vi "FFT-Rotate.vi"() -> ()   [LabVIEW 2014]
doc: "Use this template to build a VI to use as a subVI."
uses:
  <vilib>/vision/NI_Vision_Development_Module.lvlib
panel:
  out "IF(u,v)I 3":T1(plugin-control)
  out "IF(u,v)I 2":T1(plugin-control)
  out "Rotated":T1(plugin-control)
  out "IF(u,v)I":T1(plugin-control)
  out "Src":T1(plugin-control)
  # ":: MVi Framework V1.0 ::\nAuthor:Gaoke Yang\nEmail: gaoke.yang@yahoo.com\nWeb: www.mvicontrol.com\nCopyright (C) 2015, MVI Technologies All Rights Reserved"
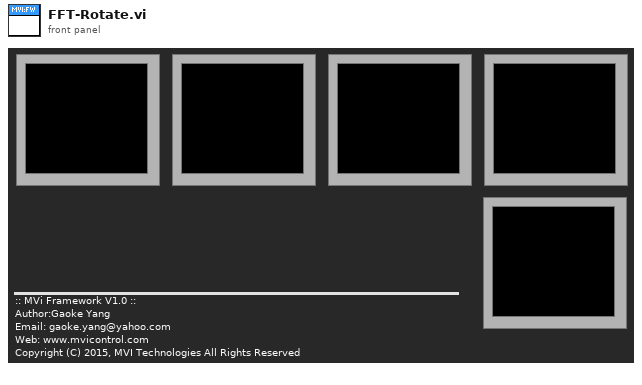
[diagram p1: front panel]
types:
  T1 = typedef "IMAQ Image.ctl" = refnum<image>
  T2 = enum32{"Real", "Imaginary", "Magnitude", "Phase"}
  T3 = typedef "Image Type" = u32
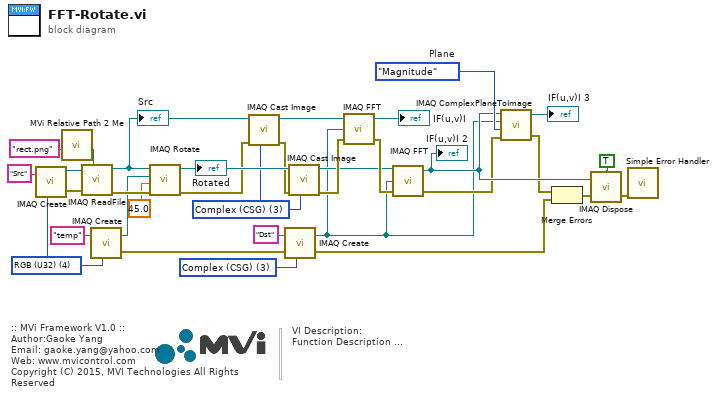
[diagram p0: block diagram]
diagram:
  w7 = T2."Magnitude"  # Plane
  w8 = T3 4 items=["Grayscale (U8)", "Grayscale (I16)", "Grayscale (SGL)", "Complex (CSG)", "RGB (U32)", "HSL (U32)", "RGB (U64)", "Grayscale (U16)"] ("Image Type")
  w16 = T3 3 items=["Grayscale (U8)", "Grayscale (I16)", "Grayscale (SGL)", "Complex (CSG)", "RGB (U32)", "HSL (U32)", "RGB (U64)", "Grayscale (U16)"] ("Image Type")
  w17 = T3 3 items=["Grayscale (U8)", "Grayscale (I16)", "Grayscale (SGL)", "Complex (CSG)", "RGB (U32)", "HSL (U32)", "RGB (U64)", "Grayscale (U16)"] ("Image Type")
  # "VI Description:\nFunction Description ..."
  # ":: MVi Framework V1.0 ::\nAuthor:Gaoke Yang\nEmail: gaoke.yang@yahoo.com\nWeb: www.mvicontrol.com\nCopyright (C) 2015, MVI Technologies All Rights Reserved"
  n1 = call "IMAQ Create"("Image Name"="Src" ("name or relative path"), "Image Type"=w8) -> ("New Image"=w30:T1, "error out"=w29:errorcluster)  [unwired: 2 in, 1 out]
  n2 = call "MVi Relative Path 2 Me.vi"("Relative Path"="rect.png" ("name or relative path")) -> ("Appended Dir"=w26:path)  [unwired: 5 in, 1 out]
  n3 = call "IMAQ ReadFile"("File Path"=w26, "error in (no error)"=w29, "Image"=w30) -> ("error out"=w25:errorcluster, "Image Out"=w22:T1)  [unwired: 4 in, 3 out]
  "Src" <- w22
  n4 = call "IMAQ Create"("Image Name"="temp" ("name or relative path"), "Image Type"=w8) -> ("New Image"=w12:T1, "error out"=w11:errorcluster)  [unwired: 2 in, 1 out]
  n5 = call "IMAQ Rotate"("error in (no error)"=w25, "Angle (degrees)"=sgl 45.0, "Image Dst"=w12, "Image Src"=w22) -> ("error out"=w10:errorcluster, "Image Dst Out"=w23:T1)  [unwired: 6 in]
  "Rotated" <- w23
  n6 = call "IMAQ Cast Image"("Image Type"=w17, "error in (no error)"=w10, "Image Src"=w22) -> ("error out"=w9:errorcluster, "Image Dst Out"=w18:T1)  [unwired: 7 in]
  n7 = call "IMAQ Create"("Image Name"="Dst" ("name or relative path"), "Image Type"=w16, "error in (no error)"=w11) -> ("New Image"=w1:T1, "error out"=w19:errorcluster)  [unwired: 1 in, 1 out]
  n8 = call "IMAQ Cast Image"("Image Type"=w17, "error in (no error)"=w9, "Image Src"=w23) -> ("error out"=w21:errorcluster, "Image Dst Out"=w14:T1)  [unwired: 7 in]
  n9 = call "IMAQ FFT"("error in (no error)"=w21, "Image Dst"=w1, "Image Src"=w18) -> ("error out"=w15:errorcluster, "Image Dst Out"=→"IF(u,v)I":T1)  [unwired: 1 in]
  n10 = call "IMAQ FFT"("error in (no error)"=w15, "Image Dst"=w1, "Image Src"=w14) -> ("error out"=w3:errorcluster, "Image Dst Out"=w4:T1)  [unwired: 1 in]
  "IF(u,v)I 2" <- w4
  n11 = call "IMAQ ComplexPlaneToImage"("error in (no error)"=w3, "Plane"=w7, "Image Dst"=w1, "Image Src"=w4) -> ("error out"=w2:errorcluster, "Image Dst Out"=→"IF(u,v)I 3":T1)  [unwired: 1 in]
  n12 = Merge Errors(w2, w19) -> (w20:errorcluster)
  n13 = call "IMAQ Dispose"("All Images? (No)"=TRUE, "Image"=w4, "error in (no error)"=w20) -> ("error out"=w31:errorcluster)  [unwired: 3 out]
  n14 = call <vilib>:"Simple Error Handler.vi"("error in (no error)"=w31) -> ()  [unwired: 1 in, 8 out]
